vi "DeleteFakeStatusFrom_DotMatrix1.vi"(2 "error IN":errorcluster, 3 "[IN] Source Matrix":i16[][](array[numeric])) -> (0 "error OUT":errorcluster, 1 "[OUT] Filtered Dot Matrix":i16[][](array[numeric]))   [LabVIEW 2013]
doc: "Delete all statuses \"-1\" of removed displacements"
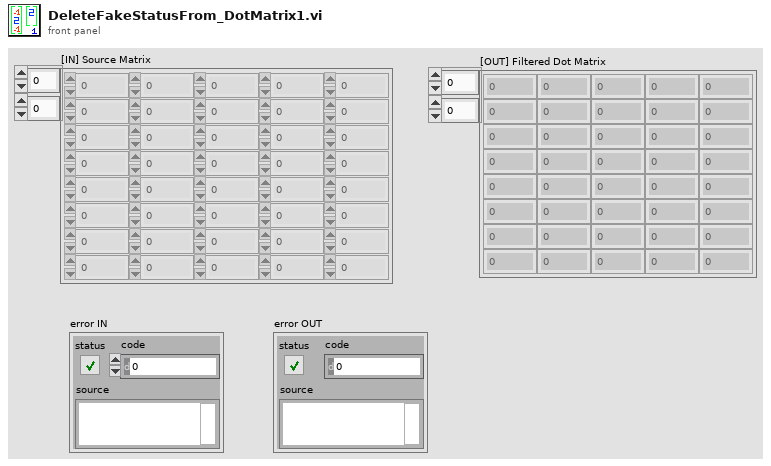
[diagram p1: front panel]
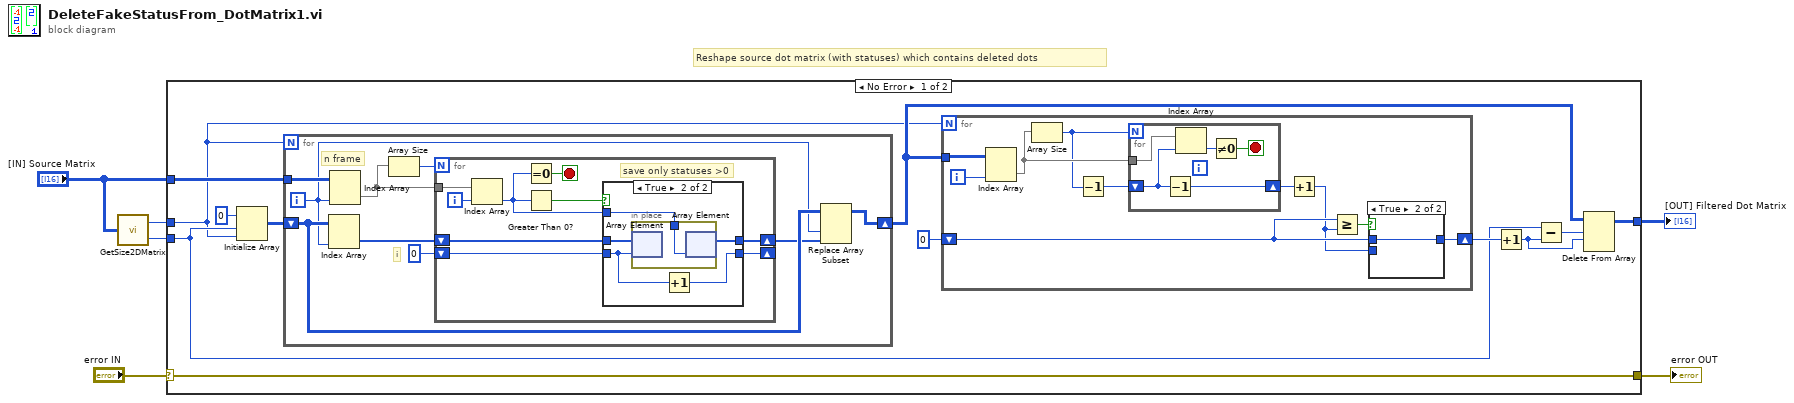
[diagram p0: block diagram]
diagram:
  # "Reshape source dot matrix (with statuses) which contains deleted dots"
  n1 = call "GetSize2DMatrix.vi"("Array IN (2D)"="[IN] Source Matrix") -> ("# Cols"=w3:i32, "# Rows"=w5:i32)
  n2 = case shown="No Error" "error IN" {
    selector: "error IN" -> [w7 w63]
    tunnel: "[IN] Source Matrix" -> [w17 w62]
    tunnel: w5 -> [w11 _]
    tunnel: [w9 w62] -> w4
    tunnel: w3 -> [w8 _]
    tunnel: [w7 w63] -> w1
    frame No Error {
      n3 = Initialize Array(i16 0 ("element"), w11, w8) -> (w16:i16[][])
      n4 = for {
        N: w8 -> [_]
        tunnel: w17 -> [w44]
        shift-right: [w41] -> w10
        shift-left: w16 -> [w42]
        i -> [w40]
        # "i"
        # "n frame"
        n5 = Index Array(array=w42, index (col)=w40) -> (element=w38:i16[])  [unwired: 1 in]
        n6 = Index Array(array=w44, index (col)=w40) -> (element=w37:i16[])  [unwired: 1 in]
        n7 = Array Size(array=w37) -> (size(s)=w36:i32)
        n8 = for {
          N: w36 -> [_]
          tunnel: w37 -> [w49]
          shift-right: [w50] -> w39
          shift-left: w38 -> [w53]
          shift-right: [w51] -> _
          shift-left: 0 -> [w52]
          i -> [w48]
          stop <- w47 stop-if-true
          # "save only statuses >0"
          n9 = Index Array(array=w49, index=w48) -> (element=w45:i16)
          n10 = Equal To 0?(x=w45) -> (x = 0?=w47:bool)
          n11 = Greater Than 0?(x=w45) -> (x > 0?=w46:bool)
          n12 = case shown="True" w46 {
            tunnel: w53 -> [w55 w59]
            tunnel: w52 -> [w54 w58]
            tunnel: [w54 w60] -> w51
            tunnel: [w55 w56] -> w50
            tunnel: w45 -> [_ w57]
            frame False {
            }
            frame True {
              n13 = in-place {
                in-place-border: w57 -> [w61]
                n14 = in-place-array #1(w59, w58) -> ()  [unwired: 1 out]
                n15 = in-place-array #1(w61) -> (w56:i16[])  [unwired: 1 out]
              }
              n16 = Increment(x=w58) -> (x+1=w60:i32)
            }
          }
        }
        n17 = Replace Array Subset(array=w42, new element=w39, index (col)=w40) -> (w41:i16[][])  [unwired: 1 in]
      }
      n18 = for {
        N: w8 -> [_]
        tunnel: w10 -> [w28]
        shift-right: [w23] -> w12
        shift-left: 0 -> [w24]
        i -> [w27]
        n19 = Index Array(array=w28, index (col)=w27) -> (element=w26:i16[])  [unwired: 1 in]
        n20 = Array Size(array=w26) -> (size(s)=w19:i32)
        n21 = Decrement(x=w19) -> (x-1=w22:i32)
        n22 = for {
          N: w19 -> [_]
          tunnel: w26 -> [w35]
          shift-right: [w33] -> w21
          shift-left: w22 -> [w31]
          stop <- w32 stop-if-true
          n23 = Decrement(x=w31) -> (x-1=w33:i32)
          n24 = Index Array(array=w35, index=w31) -> (element=w34:i16)
          n25 = Not Equal To 0?(x=w34) -> (x != 0?=w32:bool)
        }
        n26 = Increment(x=w21) -> (x+1=w20:i32)
        n27 = Greater Or Equal?(x=w24, y=w20) -> (x >= y?=w25:bool)
        n28 = case shown="True" w25 {
          tunnel: w24 -> [_ w30]
          tunnel: [w29 w30] -> w23
          tunnel: w20 -> [w29 _]
          frame False {
          }
          frame True {
          }
        }
      }
      n29 = Increment(x=w12) -> (x+1=w13:i32)
      n30 = Subtract(x=w11, y=w13) -> (x-y=w14:i32)
      n31 = Delete From Array(array=w10, length=w14, index (row)=w13) -> (array with subset deleted=w9:i16[][])  [unwired: 1 in, 1 out]
    }
    frame Error {
    }
  }
  "[OUT] Filtered Dot Matrix" <- w4
  "error OUT" <- w1
